vi "Generate_LoRa_wave.vi"() -> ()   [LabVIEW 2020]
uses:
  <instrlib>/Rohde&Schwarz RF Signal Generator/Rohde&Schwarz RF Signal Generator.lvlib
panel:
  out "error out":errorcluster
  in  "Spreading Factor (Spreading Factor 7)":i32(ring)=1 items=["Spreading Factor 6", "Spreading Factor 7", "Spreading Factor 8", "Spreading Factor 9", "Spreading Factor 10", "Spreading Factor 11", "Spreading Factor 12"]
  in  "Coding Rate (Coding Rate 1)":i32(ring)=1 items=["Coding Rate 0", "Coding Rate 1", "Coding Rate 2", "Coding Rate 3", "Coding Rate 4"]
  in  "Oversampling (4)":i32=4
  in  "Idle Interval (100.0e-6)":dbl=0.0001 format="%^.3e"
  in  "Sample Rate Variation (1.0e6)":dbl=1000000.0 format="%^.3e"
  in  "Sequence Length (1)":i32=1
  in  "Bandwidth (BW125)":i32(ring)=7 items=["BW7", "BW10", "BW15", "BW20", "BW31", "BW41", "BW62", "BW125", "BW250", "BW500"]
  in  "Enabled LoRa":bool caption="Enabled (Off)"
  in  "VISA resource name":refnum<visa-resource-name>
  in  "Instrument Name (\"instr\")":string="instr"
  in  "Address (\"192.168.1.1\")":string="192.168.1.1"
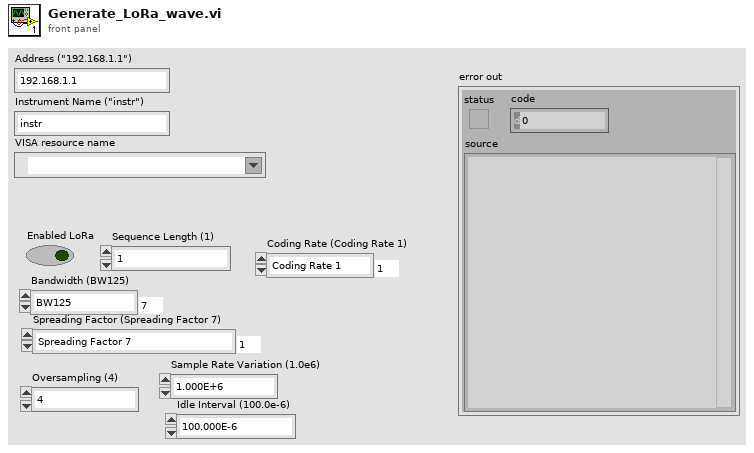
[diagram p1: front panel]
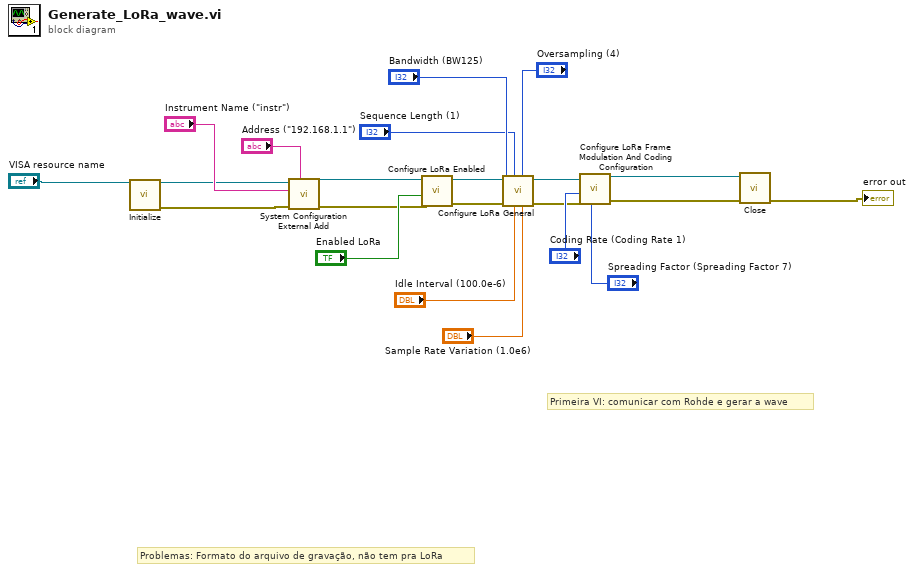
[diagram p0: block diagram]
diagram:
  # "Primeira VI: comunicar com Rohde e gerar a wave"
  # "Problemas: Formato do arquivo de gravação, não tem pra LoRa"
  n1 = call <instrlib>:"Initialize.vi"("VISA resource name"="VISA resource name") -> ("VISA resource name out"=w5:refnum<visa-resource-name>, "error out"=w4:errorcluster)  [unwired: 13 in]
  n2 = call <instrlib>:"System Configuration External Add.vi"("Address (\"192.168.1.1\")"="Address (\"192.168.1.1\")", "error in (no error)"=w4, "Instrument Name (\"instr\")"="Instrument Name (\"instr\")", "VISA resource name"=w5) -> ("error out"=w9:errorcluster, "VISA resource name out"=w19:refnum<visa-resource-name>)  [unwired: 6 in]
  n3 = call <instrlib>:"Configure LoRa Enabled.vi"("error in (no error)"=w9, "Enabled (Off)"="Enabled LoRa", "VISA resource name"=w19) -> ("error out"=w8:errorcluster, "VISA resource name out"=w18:refnum<visa-resource-name>)  [unwired: 7 in]
  n4 = call <instrlib>:"Configure LoRa General.vi"("Sample Rate Variation (1.0e6)"="Sample Rate Variation (1.0e6)", "Oversampling (4)"="Oversampling (4)", "Sequence Length (1)"="Sequence Length (1)", "Idle Interval (100.0e-6)"="Idle Interval (100.0e-6)", "error in (no error)"=w8, "Bandwidth (BW125)"="Bandwidth (BW125)", "VISA resource name"=w18) -> ("error out"=w7:errorcluster, "VISA resource name out"=w17:refnum<visa-resource-name>)  [unwired: 3 in]
  n5 = call <instrlib>:"Configure LoRa Frame Modulation And Coding Configuration.vi"("Spreading Factor (Spreading Factor 7)"="Spreading Factor (Spreading Factor 7)", "error in (no error)"=w7, "Coding Rate (Coding Rate 1)"="Coding Rate (Coding Rate 1)", "VISA resource name"=w17) -> ("error out"=w3:errorcluster, "VISA resource name out"=w2:refnum<visa-resource-name>)  [unwired: 6 in]
  n6 = call <instrlib>:"Close.vi"("error in (no error)"=w3, "VISA resource name"=w2) -> ("error out"=→"error out":errorcluster)  [unwired: 9 in]
